vi "DynamicCallVI-Open Frant Panel.vi"(8 "error in (no error)":errorcluster, 10 "name or relative path":string, 11 "base path":path) -> (0 "error out":errorcluster, 3 "appended path":path)   [LabVIEW 2021]
doc: "dynamic call a vi, is used in the launcher, usually.\n2014-11-04 10:18:58\n蒋松\njiangsong@outlook.com"
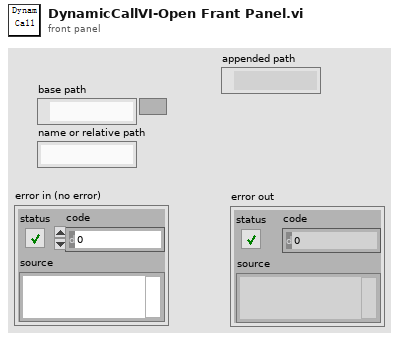
[diagram p1: front panel]
types:
  T1 = enum32{"Invalid", "Standard", "Closed", "Hidden", "Minimized", "Maximized"}
  T2 = enum32{"Bad", "Idle", "Run top level", "Running"}
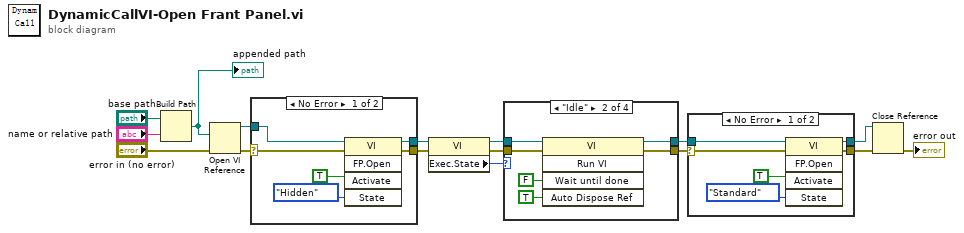
[diagram p0: block diagram]
diagram:
  n1 = Build Path(base path="base path", name or relative path="name or relative path") -> (appended path=w16:path)
  "appended path" <- w16
  n2 = Open VI Reference(vi path=w16, error in (no error)="error in (no error)") -> (vi reference=w14:refnum<vi>, error out=w15:errorcluster)  [unwired: 4 in]
  n3 = case shown="No Error" w15 {
    selector: w15 -> [w17 w23]
    tunnel: [w20 w23] -> w13
    tunnel: w14 -> [w19 w24]
    tunnel: [w18 w24] -> w9
    frame No Error {
      n4 = invoke class="VI" method="FP.Open"(reference=w19, error in=w17, "Activate"=TRUE, "State"=T1."Hidden") -> (reference out=w18:refnum<vi>, error out=w20:errorcluster)  [unwired: 1 in, 3 out]
    }
    frame Error {
    }
  }
  n5 = property class="VI"(reference=w9, error in=w13) -> (reference out=w11:refnum<vi>, error out=w10:errorcluster, "Exec.State"=w12:T2)
  n6 = case shown="\"Idle\"" w12 {
    tunnel: w11 -> [w26 w30 w34 w36]
    tunnel: w10 -> [w25 w29 w33 w35]
    tunnel: [w26 w28 w34 w36] -> w8
    tunnel: [w25 w27 w33 w35] -> w6
    frame "Bad", Default {
    }
    frame "Idle" {
      n7 = invoke class="VI" method="Run VI"(reference=w30, error in=w29, "Wait until done"=FALSE ("Wait Until Done"), "Auto Dispose Ref"=TRUE ("Auto Dispose Reference")) -> (reference out=w28:refnum<vi>, error out=w27:errorcluster)  [unwired: 1 in, 3 out]
    }
    frame "Run top level" {
    }
    frame "Running" {
    }
  }
  n8 = case shown="No Error" w6 {
    selector: w6 -> [w37 w43]
    tunnel: [w40 w43] -> w5
    tunnel: w8 -> [w39 w44]
    tunnel: [w38 w44] -> w7
    frame No Error {
      n9 = invoke class="VI" method="FP.Open"(reference=w39, error in=w37, "Activate"=TRUE, "State"=T1."Standard") -> (reference out=w38:refnum<vi>, error out=w40:errorcluster)  [unwired: 1 in, 3 out]
    }
    frame Error {
    }
  }
  n10 = Close Reference(reference=w7, error in (no error)=w5) -> (error out=→"error out":errorcluster)
